vi "VCI_BOARD_INFO_CONVERT.vi"(1 "VCI_BOARD_INFO":T2) -> (0 "VCI_BOARD_INFO_1":T1)   [LabVIEW 2018, in "ControlCan.lvlib"]
uses:
  ControlCan.lvlib
  VCI_BOARD_INFO.ctl
  VCI_BOARD_INFO_1.ctl
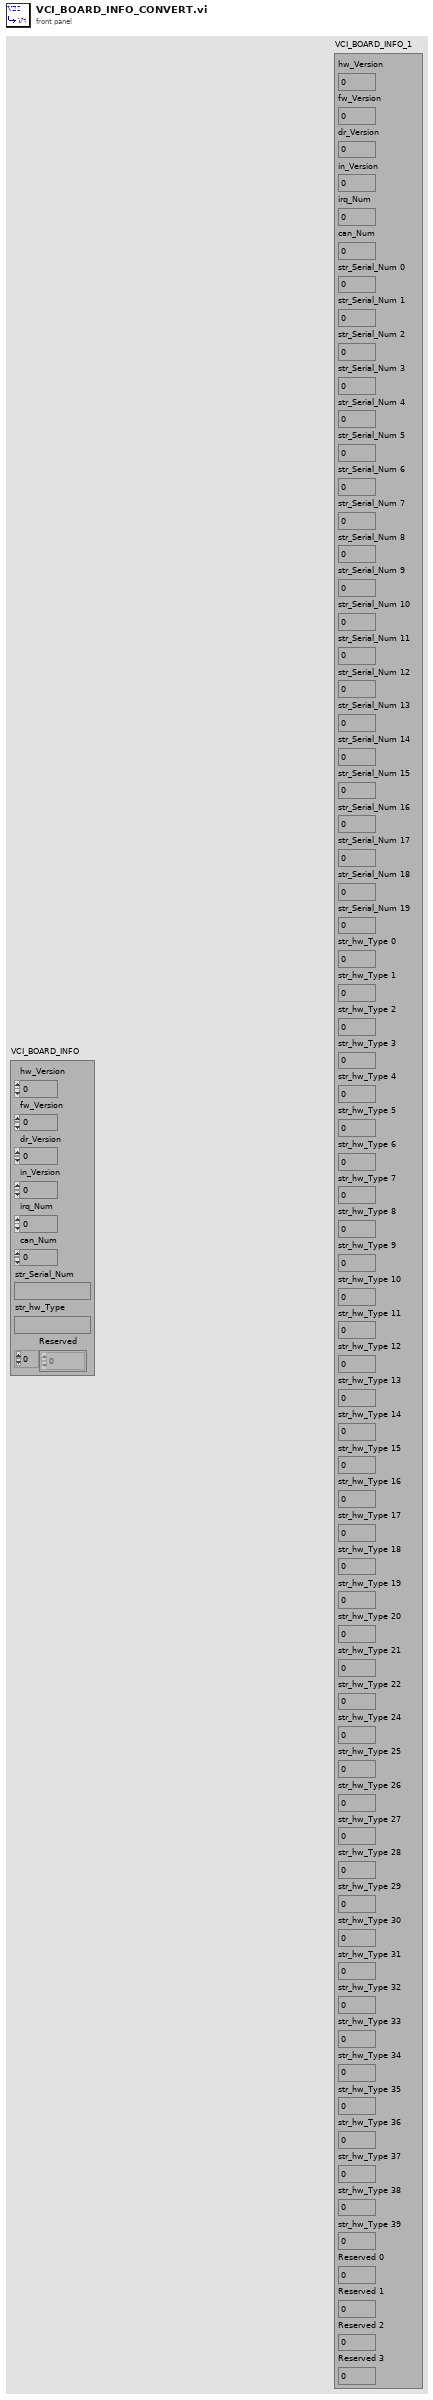
[diagram p1: front panel]
types:
  T1 = typedef "ControlCAN.lvlib/VCI_BOARD_INFO_1.ctl" = cluster{"hw_Version":u16, "fw_Version":u16, "dr_Version":u16, "in_Version":u16, "irq_Num":u16, "can_Num":u8, "str_Serial_Num 0":u8, "str_Serial_Num 1":u8, "str_Serial_Num 2":u8, "str_Serial_Num 3":u8, "str_Serial_Num 4":u8, "str_Serial_Num 5":u8, "str_Serial_Num 6":u8, "str_Serial_Num 7":u8, "str_Serial_Num 8":u8, "str_Serial_Num 9":u8, "str_Serial_Num 10":u8, "str_Serial_Num 11":u8, "str_Serial_Num 12":u8, "str_Serial_Num 13":u8, "str_Serial_Num 14":u8, "str_Serial_Num 15":u8, "str_Serial_Num 16":u8, "str_Serial_Num 17":u8, "str_Serial_Num 18":u8, "str_Serial_Num 19":u8, "str_hw_Type 0":u8, "str_hw_Type 1":u8, "str_hw_Type 2":u8, "str_hw_Type 3":u8, "str_hw_Type 4":u8, "str_hw_Type 5":u8, "str_hw_Type 6":u8, "str_hw_Type 7":u8, "str_hw_Type 8":u8, "str_hw_Type 9":u8, "str_hw_Type 10":u8, "str_hw_Type 11":u8, "str_hw_Type 12":u8, "str_hw_Type 13":u8, "str_hw_Type 14":u8, "str_hw_Type 15":u8, "str_hw_Type 16":u8, "str_hw_Type 17":u8, "str_hw_Type 18":u8, "str_hw_Type 19":u8, "str_hw_Type 20":u8, "str_hw_Type 21":u8, "str_hw_Type 22":u8, "str_hw_Type 24":u8, "str_hw_Type 25":u8, "str_hw_Type 26":u8, "str_hw_Type 27":u8, "str_hw_Type 28":u8, "str_hw_Type 29":u8, "str_hw_Type 30":u8, "str_hw_Type 31":u8, "str_hw_Type 32":u8, "str_hw_Type 33":u8, "str_hw_Type 34":u8, "str_hw_Type 35":u8, "str_hw_Type 36":u8, "str_hw_Type 37":u8, "str_hw_Type 38":u8, "str_hw_Type 39":u8, "Reserved 0":u8, "Reserved 1":u8, "Reserved 2":u8, "Reserved 3":u8}
  T2 = typedef "ControlCAN.lvlib/VCI_BOARD_INFO.ctl" = cluster{"hw_Version":u16, "fw_Version":u16, "dr_Version":u16, "in_Version":u16, "irq_Num":u16, "can_Num":u8, "str_Serial_Num":string, "str_hw_Type":string, "Reserved":u8[]}
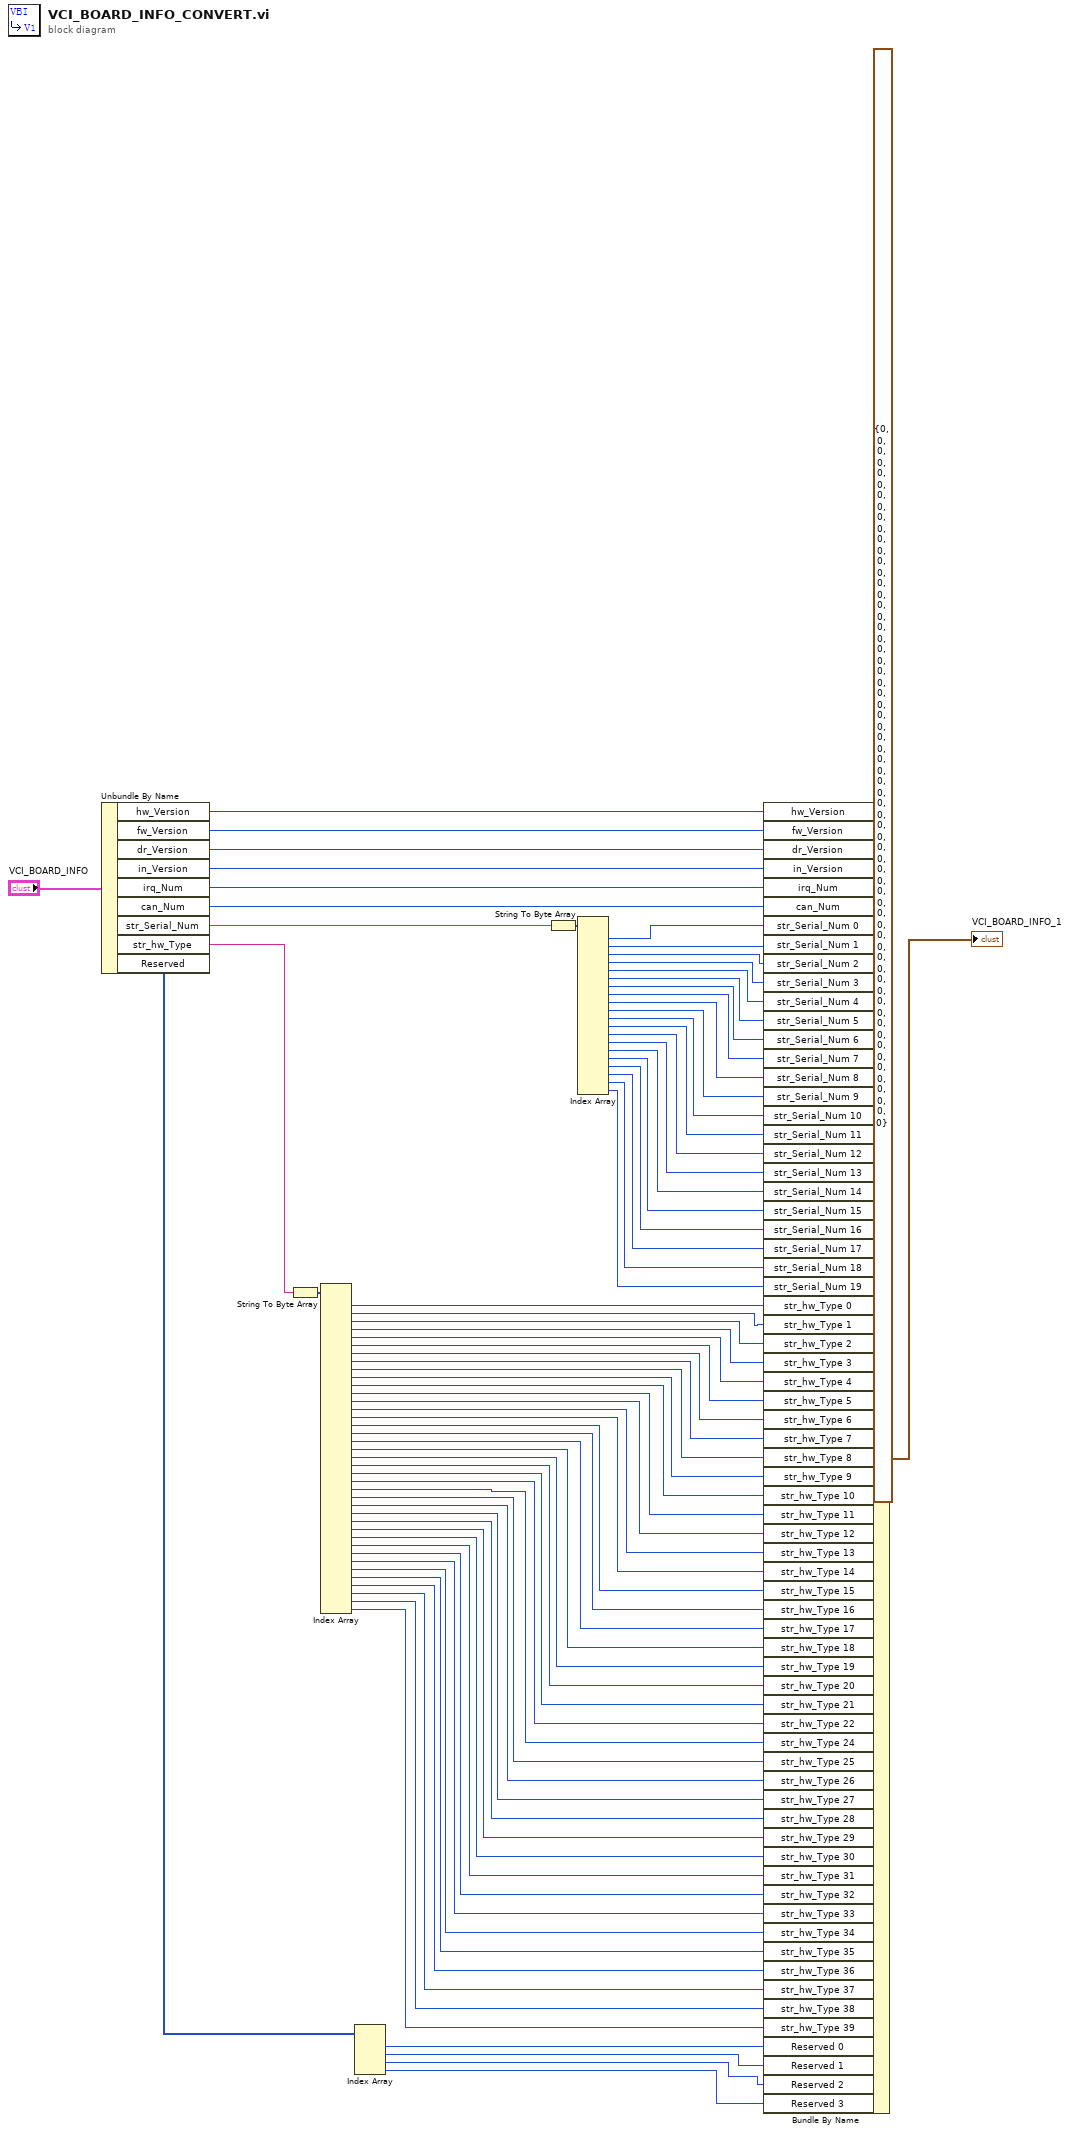
[diagram p0: block diagram]
diagram:
  n1 = Unbundle By Name("VCI_BOARD_INFO") -> ("hw_Version"=w75:u16, "fw_Version"=w74:u16, "dr_Version"=w73:u16, "in_Version"=w72:u16, "irq_Num"=w71:u16, "can_Num"=w70:u8, "str_Serial_Num"=w69:string, "str_hw_Type"=w46:string, "Reserved"=w5:u8[])
  n2 = String To Byte Array(string=w46) -> (unsigned byte array=w45:u8[])
  n3 = Index Array(array=w45) -> (element #1=w44:u8, element #2=w43:u8, element #3=w42:u8, element #4=w41:u8, element #5=w40:u8, element #6=w39:u8, element #7=w38:u8, element #8=w37:u8, element #9=w36:u8, element #10=w35:u8, element #11=w34:u8, element #12=w33:u8, element #13=w32:u8, element #14=w31:u8, element #15=w30:u8, element #16=w29:u8, element #17=w28:u8, element #18=w27:u8, element #19=w26:u8, element #20=w25:u8, element #21=w24:u8, element #22=w23:u8, element #23=w22:u8, element #24=w21:u8, element #25=w20:u8, element #26=w19:u8, element #27=w18:u8, element #28=w17:u8, element #29=w16:u8, element #30=w15:u8, element #31=w14:u8, element #32=w13:u8, element #33=w12:u8, element #34=w11:u8, element #35=w10:u8, element #36=w9:u8, element #37=w8:u8, element #38=w7:u8, element #39=w6:u8)  [unwired: 39 in]
  n4 = Index Array(array=w5) -> (element #1=w4:u8, element #2=w3:u8, element #3=w2:u8, element #4=w1:u8)  [unwired: 4 in]
  n5 = String To Byte Array(string=w69) -> (unsigned byte array=w68:u8[])
  n6 = Index Array(array=w68) -> (element #1=w67:u8, element #2=w66:u8, element #3=w65:u8, element #4=w64:u8, element #5=w63:u8, element #6=w62:u8, element #7=w61:u8, element #8=w60:u8, element #9=w58:u8, element #10=w57:u8, element #11=w56:u8, element #12=w55:u8, element #13=w54:u8, element #14=w53:u8, element #15=w52:u8, element #16=w51:u8, element #17=w50:u8, element #18=w49:u8, element #19=w48:u8, element #20=w47:u8)  [unwired: 20 in]
  n7 = Bundle By Name(cluster=T1 {"hw_Version"=0, "fw_Version"=0, "dr_Version"=0, "in_Version"=0, "irq_Num"=0, "can_Num"=0, "str_Serial_Num 0"=0, "str_Serial_Num 1"=0, "str_Serial_Num 2"=0, "str_Serial_Num 3"=0, "str_Serial_Num 4"=0, "str_Serial_Num 5"=0, "str_Serial_Num 6"=0, "str_Serial_Num 7"=0, "str_Serial_Num 8"=0, "str_Serial_Num 9"=0, "str_Serial_Num 10"=0, "str_Serial_Num 11"=0, "str_Serial_Num 12"=0, "str_Serial_Num 13"=0, "str_Serial_Num 14"=0, "str_Serial_Num 15"=0, "str_Serial_Num 16"=0, "str_Serial_Num 17"=0, "str_Serial_Num 18"=0, "str_Serial_Num 19"=0, "str_hw_Type 0"=0, "str_hw_Type 1"=0, "str_hw_Type 2"=0, "str_hw_Type 3"=0, "str_hw_Type 4"=0, "str_hw_Type 5"=0, "str_hw_Type 6"=0, "str_hw_Type 7"=0, "str_hw_Type 8"=0, "str_hw_Type 9"=0, "str_hw_Type 10"=0, "str_hw_Type 11"=0, "str_hw_Type 12"=0, "str_hw_Type 13"=0, "str_hw_Type 14"=0, "str_hw_Type 15"=0, "str_hw_Type 16"=0, "str_hw_Type 17"=0, "str_hw_Type 18"=0, "str_hw_Type 19"=0, "str_hw_Type 20"=0, "str_hw_Type 21"=0, "str_hw_Type 22"=0, "str_hw_Type 24"=0, "str_hw_Type 25"=0, "str_hw_Type 26"=0, "str_hw_Type 27"=0, "str_hw_Type 28"=0, "str_hw_Type 29"=0, "str_hw_Type 30"=0, "str_hw_Type 31"=0, "str_hw_Type 32"=0, "str_hw_Type 33"=0, "str_hw_Type 34"=0, "str_hw_Type 35"=0, "str_hw_Type 36"=0, "str_hw_Type 37"=0, "str_hw_Type 38"=0, "str_hw_Type 39"=0, "Reserved 0"=0, "Reserved 1"=0, "Reserved 2"=0, "Reserved 3"=0} ("VCI_BOARD_INFO_1"), "hw_Version"=w75, "fw_Version"=w74, "dr_Version"=w73, "in_Version"=w72, "irq_Num"=w71, "can_Num"=w70, "str_Serial_Num 0"=w67, "str_Serial_Num 1"=w66, "str_Serial_Num 2"=w65, "str_Serial_Num 3"=w64, "str_Serial_Num 4"=w63, "str_Serial_Num 5"=w62, "str_Serial_Num 6"=w61, "str_Serial_Num 7"=w60, "str_Serial_Num 8"=w58, "str_Serial_Num 9"=w57, "str_Serial_Num 10"=w56, "str_Serial_Num 11"=w55, "str_Serial_Num 12"=w54, "str_Serial_Num 13"=w53, "str_Serial_Num 14"=w52, "str_Serial_Num 15"=w51, "str_Serial_Num 16"=w50, "str_Serial_Num 17"=w49, "str_Serial_Num 18"=w48, "str_Serial_Num 19"=w47, "str_hw_Type 0"=w44, "str_hw_Type 1"=w43, "str_hw_Type 2"=w42, "str_hw_Type 3"=w41, "str_hw_Type 4"=w40, "str_hw_Type 5"=w39, "str_hw_Type 6"=w38, "str_hw_Type 7"=w37, "str_hw_Type 8"=w36, "str_hw_Type 9"=w35, "str_hw_Type 10"=w34, "str_hw_Type 11"=w33, "str_hw_Type 12"=w32, "str_hw_Type 13"=w31, "str_hw_Type 14"=w30, "str_hw_Type 15"=w29, "str_hw_Type 16"=w28, "str_hw_Type 17"=w27, "str_hw_Type 18"=w26, "str_hw_Type 19"=w25, "str_hw_Type 20"=w24, "str_hw_Type 21"=w23, "str_hw_Type 22"=w22, "str_hw_Type 24"=w21, "str_hw_Type 25"=w20, "str_hw_Type 26"=w19, "str_hw_Type 27"=w18, "str_hw_Type 28"=w17, "str_hw_Type 29"=w16, "str_hw_Type 30"=w15, "str_hw_Type 31"=w14, "str_hw_Type 32"=w13, "str_hw_Type 33"=w12, "str_hw_Type 34"=w11, "str_hw_Type 35"=w10, "str_hw_Type 36"=w9, "str_hw_Type 37"=w8, "str_hw_Type 38"=w7, "str_hw_Type 39"=w6, "Reserved 0"=w4, "Reserved 1"=w3, "Reserved 2"=w2, "Reserved 3"=w1) -> (→"VCI_BOARD_INFO_1":T1)
